vi "Do This.vi"(8 "error in (no error)":errorcluster, 10 "Status Events":refnum<class "Status Events.lvclass">, 11 "VIP Uninstall in":refnum<class "VIPM Update.lvclass">) -> (0 "error out":errorcluster, 3 "VIP Uninstall out":refnum<class "VIPM Update.lvclass">)   [LabVIEW 2014, in "VIPM Update.lvclass"]
uses:
  VIPM Update.lvclass
  Classes/Status Events/Status Events.lvclass
  VIPM Update.lvclass/VIPM Update.ctl
  <vilib>/Utility/error.llb/DialogType.ctl
  Classes/Job/Job.lvclass/Job.ctl
  Classes/Job/Job.lvclass
  <vilib>/JKI/VIPM API/VIPM API_vipm_api.lvlib
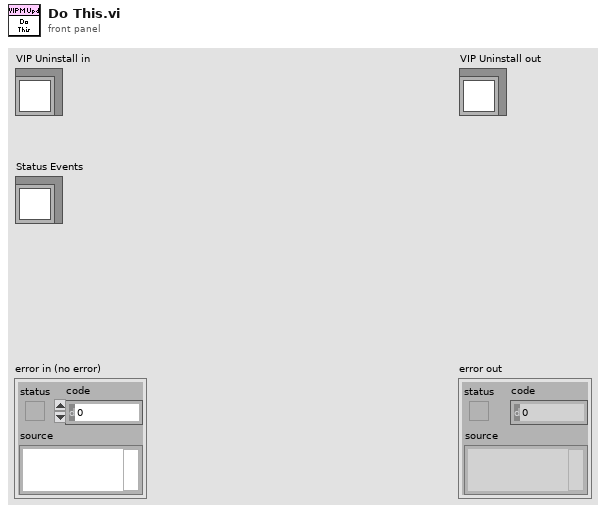
[diagram p1: front panel]
types:
  T1 = typedef "DialogType.ctl" = u16
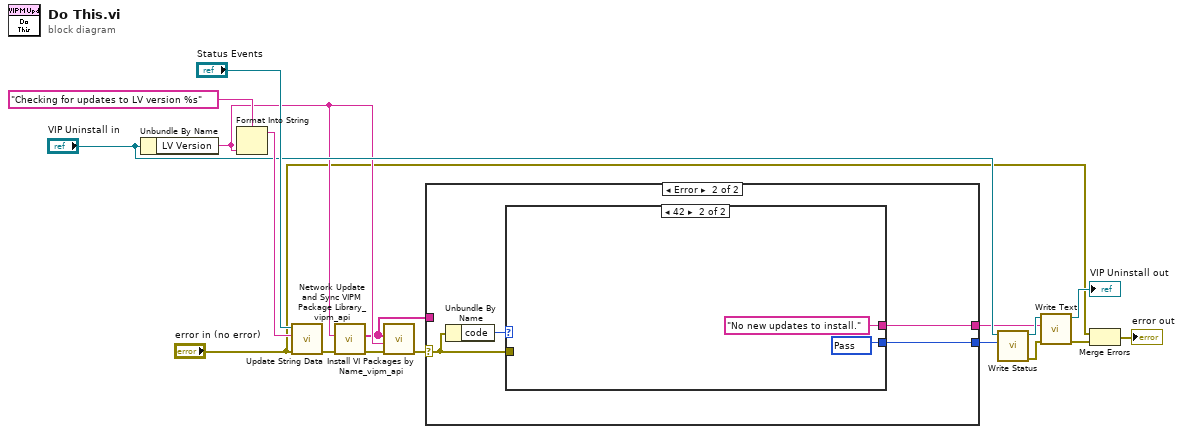
[diagram p0: block diagram]
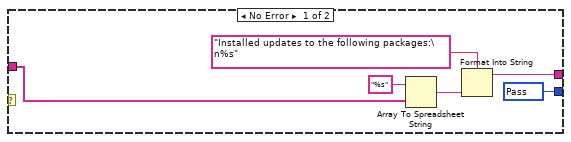
[diagram p2: hidden frame]
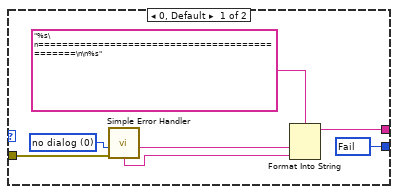
[diagram p3: hidden frame]
diagram:
  n1 = Unbundle By Name("VIP Uninstall in") -> ("LV Version"=w6:string)
  n2 = Format Into String(format string="Checking for updates to LV version %s", w6) -> (resulting string=w15:string)  [unwired: 2 in, 1 out]
  n3 = call "Update String Data.vi"("error in (no error)"="error in (no error)", "String Data"=w15, "Status Updater in"="Status Events") -> ("error out"=w8:errorcluster)  [unwired: 7 in, 1 out]
  n4 = call <vilib>:"Network Update and Sync VIPM Package Library_vipm_api.vi"("error in (no error)"=w8, "LabVIEW Version"=w6) -> ("error out"=w7:errorcluster, "New Package Updates"=w4:string[])  [unwired: 8 in]
  n5 = call <vilib>:"Install VI Packages by Name_vipm_api.vi"("error in (no error)"=w7, "LabVIEW Version"=w6, "Package Names to Install []"=w4) -> ("error out"=w5:errorcluster)  [unwired: 8 in]
  n6 = case shown="Error" w5 {
    selector: w5 -> [_ w25]
    tunnel: [w23 w27] -> w2
    tunnel: [w21 w26] -> w3
    tunnel: w4 -> [w20 _]
    frame No Error {
      w23 = u16 200 items=["Abort"=503, "Fail"=500, "Pass"=200] ("Status")
      n7 = Array To Spreadsheet String(array=w20, 3:"%s" ("format string")) -> (spreadsheet string=w19:string)  [unwired: 1 in]
      n8 = Format Into String(format string="Installed updates to the following packages:\n%s", w19) -> (resulting string=w21:string)  [unwired: 2 in, 1 out]
    }
    frame Error {
      n9 = Unbundle By Name(w25) -> ("code"=w24:i32)
      n10 = case shown="42" w24 {
        tunnel: [w34 w36] -> w27
        tunnel: [w29 "No new updates to install."] -> w26
        tunnel: w25 -> [w28 _]
        frame 0, Default {
          w30 = T1 0 items=["no dialog", "OK message", "continue or stop message", "OK message + warnings", "continue/stop + warnings"] ("type of dialog (OK msg:1)")
          w34 = u16 500 items=["Abort"=503, "Fail"=500, "Pass"=200] ("Status")
          n11 = call <vilib>:"Simple Error Handler.vi"("type of dialog (OK msg:1)"=w30, "error in (no error)"=w28) -> ("source out"=w32:string, "message"=w33:string)  [unwired: 3 in, 3 out]
          n12 = Format Into String(format string="%s\n==============================================\n\n%s", w32, w33) -> (resulting string=w29:string)  [unwired: 2 in, 1 out]
        }
        frame 42 {
          w36 = u16 200 items=["Abort"=503, "Fail"=500, "Pass"=200] ("Status")
        }
      }
    }
  }
  n13 = call "Write Status.vi"("Status"=w2, "Job in"="VIP Uninstall in") -> ("error out"=w12:errorcluster, "Job out"=w13:refnum<class "VIPM Update.lvclass">)  [unwired: 8 in]
  n14 = call "Write Text.vi"("error in (no error)"=w12, "Text"=w3, "Job in"=w13) -> ("error out"=w10:errorcluster, "Job out"=→"VIP Uninstall out":refnum<class "VIPM Update.lvclass">)  [unwired: 7 in]
  n15 = Merge Errors("error in (no error)", w10) -> (→"error out":errorcluster)
